vi "Data.idle.vi"(7 "write?":bool, 8 "error in":errorcluster, 10 "idle in":bool) -> (0 "error thru":errorcluster, 2 "idle?":bool=TRUE)   [LabVIEW 2020]
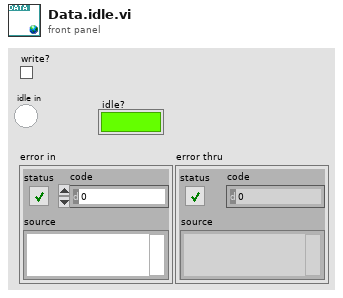
[diagram p1: front panel]
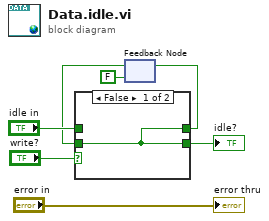
[diagram p0: block diagram]
diagram:
  n1 = feedback #1(FALSE ("idle in")) -> (w3:bool)
  n2 = case shown="False" "write?" {
    tunnel: "idle in" -> [_ w9]
    tunnel: w3 -> [w8 _]
    tunnel: [w8 w9] -> w4
    tunnel: [w8 _] -> w1
    frame False {
    }
    frame True {
    }
  }
  "idle?" <- w1
  n3 = feedback-in #1(w4) -> ()
  "error thru" <- "error in"
